vi "Read Setting Range.vi"(8 "error in (no error)":errorcluster, 10 "Operation Mode (0: Current)":u16(ring) items=["Current", "Voltage", "Resistance", "Power"], 11 "VISA resource name":refnum<visa-resource-name>) -> (0 "error out":errorcluster, 1 "Min Setting Range":dbl format="%^#_6g", 2 "Max Setting Range":dbl format="%^#_6g", 3 "VISA resource name out":refnum<visa-resource-name>)   [LabVIEW 2017, in "HH PLI Series.lvlib"]
doc: "Reads the maximum and minimum nominal setting range corresponding to the selected operation mode."
uses:
  HH PLI Series.lvlib
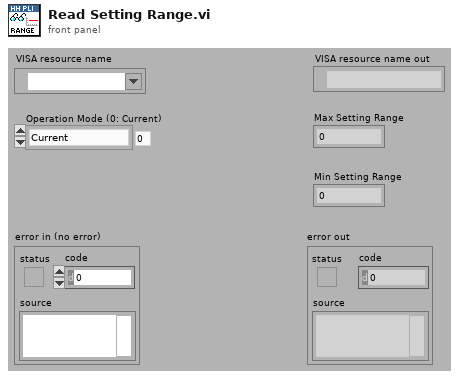
[diagram p1: front panel]
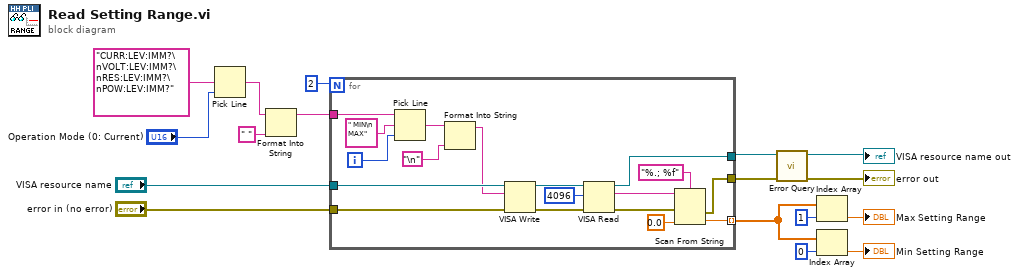
[diagram p0: block diagram]
diagram:
  n1 = Pick Line(multi-line string="CURR:LEV:IMM?\nVOLT:LEV:IMM?\nRES:LEV:IMM?\nPOW:LEV:IMM?", line index="Operation Mode (0: Current)") -> (output string=w2:string)  [unwired: 1 in]
  n2 = Format Into String(initial string=w2, " " ("string")) -> (resulting string=w1:string)  [unwired: 2 in, 1 out]
  n3 = for {
    N: 2 -> [_]
    tunnel: "VISA resource name" -> [w35]
    tunnel: "error in (no error)" -> [w34]
    tunnel: [w31] -> w11
    tunnel: [w25] -> w13
    tunnel: [w24] -> w8 mode=indexing
    tunnel: w1 -> [w18]
    i -> [w22]
    n4 = Pick Line(string ("")=w18, multi-line string=" MIN\n MAX", line index=w22) -> (output string=w20:string)
    n5 = Format Into String(initial string=w20, "\n") -> (resulting string=w21:string)  [unwired: 2 in, 1 out]
    n6 = VISA Write(VISA resource name=w35, write buffer=w21, error in (no error)=w34) -> (VISA resource name out=w33:refnum<visa-resource-name>, error out=w32:errorcluster)  [unwired: 1 out]
    n7 = VISA Read(VISA resource name=w33, byte count=u32 4096, error in (no error)=w32) -> (VISA resource name out=w31:refnum<visa-resource-name>, read buffer=w29:string, error out=w27:errorcluster)  [unwired: 1 out]
    n8 = Scan From String(format string="%.; %f", input string=w29, error in=w27, default 1=0.0 ("default value 1")) -> (error out=w25:errorcluster, output 1=w24:dbl)  [unwired: 1 in, 2 out]
  }
  n9 = call "Error Query.vi"("error in (no error)"=w13, "VISA resource name"=w11) -> ("error out"=→"error out":errorcluster, "VISA resource name out"=→"VISA resource name out":refnum<visa-resource-name>)  [unwired: 6 in, 2 out]
  n10 = Index Array(array=w8, index=1) -> (element=→"Max Setting Range":dbl)
  n11 = Index Array(array=w8, index=0) -> (element=→"Min Setting Range":dbl)
